vi "Simulateur_chinook.vi"() -> ()   [LabVIEW 2010]
panel:
  in  "FIO7 2":bool
  in  "Numérique (hz)":dbl
  out "Numeric":i32
  in  "FIO7":bool
  in  "DAC1":dbl(slide) scale=0.0..3.3
  in  "DAC0":dbl(slide) scale=0.0..3.3
  in  "FIO1":bool
  in  "FIO0":bool
  in  "FIO4":bool
  in  "FIO2":bool
  in  "FIO5":bool
  in  "FIO3":bool
  in  "FIO6":bool
  out "Error":string
  in  "Stop":bool
  # "SMT Signal Cluster (complexl).ctlUpdates DAC0 at the specified update interval in order to build time series waveforms.  The\nupdate interval is set to 20 ms by default, but can be set lower based on the execution times\ndiscussed in Section 3.1 of the U3 User's Guide.  Uses the first found U3.\n\nWith a software timed application such as this, you might be able to reduce timing jitter (caused\nby the operating system) by increasing the priority of this process (labview.exe) in Windows\nTask Manager."
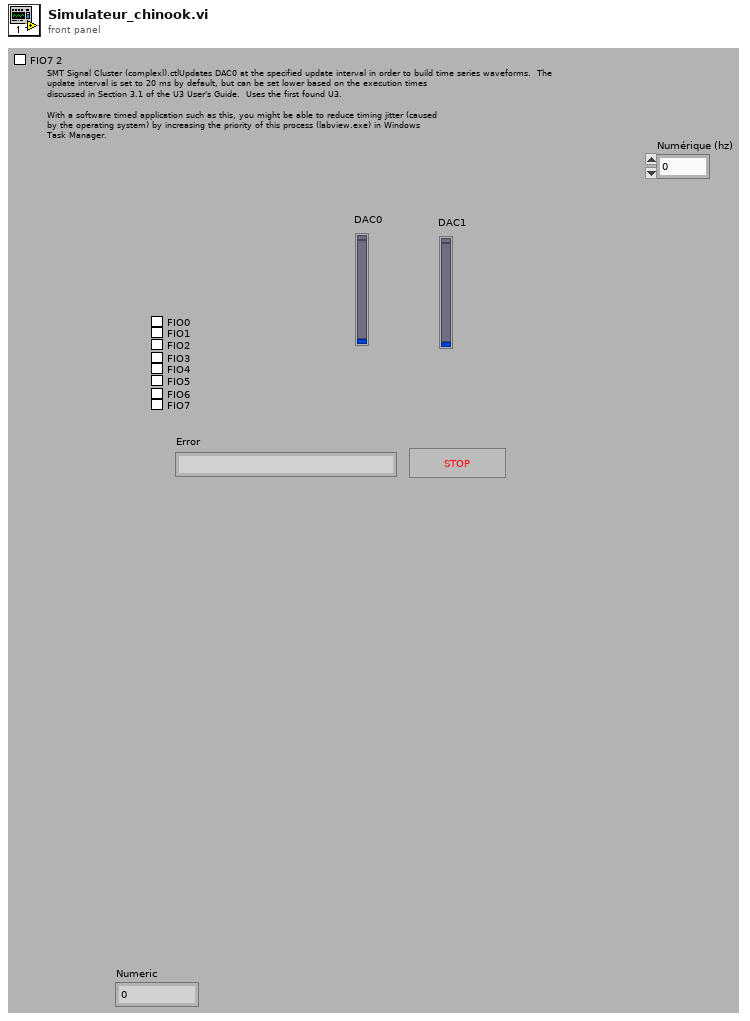
[diagram p1: front panel]
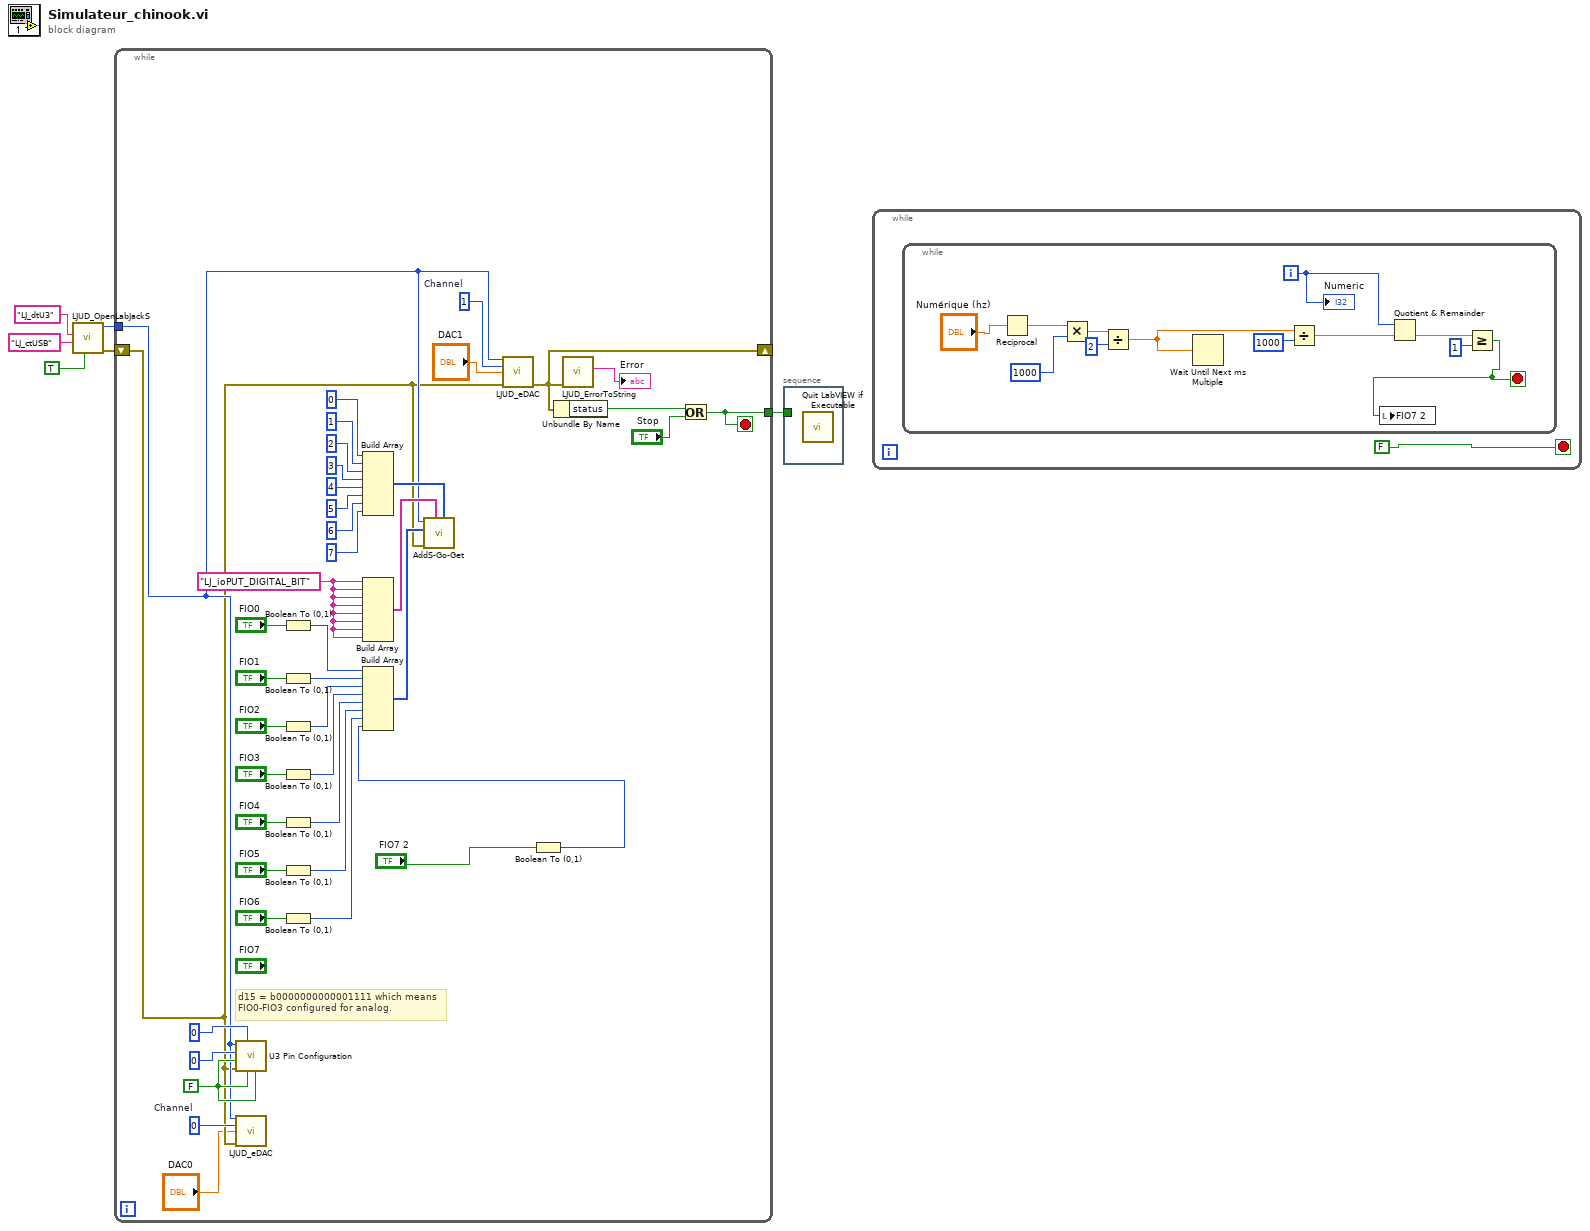
[diagram p0: block diagram]
diagram:
  n1 = call "LJUD_OpenLabJackS.vi"("FirstFound"=TRUE, "ConnectionType"="LJ_ctUSB", "DeviceType"="LJ_dtU3") -> ("error out"=w2:errorcluster, "Handle"=w1:i32)  [unwired: 6 in, 1 out]
  n2 = while {
    tunnel: w1 -> [w14]
    shift-left: w2 -> [w13]
    shift-right: [w44] -> _
    tunnel: [w9] -> w6
    stop <- w9 stop-if-true
    w15 = 0  # Channel
    w12 = "LJ_ioPUT_DIGITAL_BIT" ("IOType")
    w41 = FALSE ("Enable DAC1")
    w45 = 1  # Channel
    # "d15 = b0000000000001111 which means\nFIO0-FIO3 configured for analog."
    n3 = call "U3 Pin Configuration.vi"("Enable Counter1"=w41, "Enable Counter0"=w41, "FIO/EIO Analog Enable"=0, "error in"=w13, "Enable DAC1"=w41, "Number of Timers Enabled"=u8 0, "Handle In"=w14) -> ()  [unwired: 3 in, 2 out]
    n4 = call "LJUD_eDAC.vi"("Handle In"=w14, "Channel"=w15, "Voltage"="DAC0", "error in"=w13) -> ()  [unwired: 10 in, 2 out]
    n5 = Boolean To (0,1)(Boolean="FIO0") -> (0, 1=w16:i16)
    n6 = Boolean To (0,1)(Boolean="FIO1") -> (0, 1=w18:i16)
    n7 = Boolean To (0,1)(Boolean="FIO2") -> (0, 1=w20:i16)
    n8 = Boolean To (0,1)(Boolean="FIO3") -> (0, 1=w22:i16)
    n9 = Boolean To (0,1)(Boolean="FIO4") -> (0, 1=w24:i16)
    n10 = Boolean To (0,1)(Boolean="FIO5") -> (0, 1=w26:i16)
    n11 = Boolean To (0,1)(Boolean="FIO6") -> (0, 1=w40:i16)
    n12 = Build Array(0, 1, 2, 3, 4, 5, 6, 7) -> (w28:i32[])
    n13 = Build Array(w12, w12, w12, w12, w12, w12, w12, w12) -> (w29:string[])
    n14 = call "LJUD_eDAC.vi"("Handle In"=w14, "Channel"=w45, "Voltage"="DAC1", "error in"=w13) -> ("error out"=w44:errorcluster)  [unwired: 10 in, 1 out]
    n15 = Boolean To (0,1)(Boolean="FIO7 2") -> (0, 1=w8:i16)
    n16 = Build Array(w16, w18, w20, w22, w24, w26, w40, w8) -> (w39:i16[])
    n17 = call "AddS-Go-Get.vi"("Channels"=w28, "IOTypes"=w29, "error in"=w13, "Values Write"=w39, "Handle In"=w14) -> ()  [unwired: 4 in, 3 out]
    n18 = Unbundle By Name(w44) -> ("status"=w46:bool)
    n19 = call "LJUD_ErrorToString.vi"("error in"=w44) -> ("String"=→"Error":string)  [unwired: 10 in]
    n20 = Or(x=w46, y="Stop") -> (x .or. y?=w9:bool)
  }
  n21 = stacked-sequence {
    tunnel: w6 -> [_]
    frame #0 {
      n22 = call "Quit LabVIEW if Executable.vi"() -> ()  [unwired: 1 in]
    }
  }
  n23 = while {
    stop <- FALSE stop-if-true
    n24 = while {
      i -> [w57]
      stop <- w50 stop-if-true
      n25 = Reciprocal(x="Numérique (hz)") -> (1/x=w52:dbl)
      n26 = Multiply(x=w52, y=1000 ("Count(Ticks)")) -> (x*y=w54:dbl)
      n27 = Divide(x=w54, y=2 ("Count(Ticks)")) -> (x/y=w55:dbl)
      n28 = Wait Until Next ms Multiple(millisecond multiple=w55) -> ()  [unwired: 1 out]
      n29 = Divide(x=w55, y=1000 ("Count(Ticks)")) -> (x/y=w60:dbl)
      n30 = Quotient & Remainder(x=w57, y=w60) -> (floor(x/y)=w58:dbl)  [unwired: 1 out]
      n31 = Greater Or Equal?(x=w58, y=1 ("Count(Ticks)")) -> (x >= y?=w50:bool)
      n32 = local write "FIO7 2"(w50) -> ()
      "Numeric" <- w57
    }
  }
